vi "HW_Gantner_Search Devices in System.vi"(8 "error in":errorcluster caption="错误输入") -> (0 "error out":errorcluster caption="错误输出", 1 "Modu[] info":T7[](array[typedef]), 3 "Configuration out":T1 {"StartTime" format="%#.10f"; "dActTimeToSecondFactor" format="%#.10f"; "StartTimeToDayFactor" format="%#_10f"})   [LabVIEW 2016]
doc: "检测系统中的NI设备：\n包括机箱信息、模块信息、通道基本信息等。\n\n两种方式：\n1、配置文件中读取\n2、自动检测\n具体实现方式在配置文件中配置。"
uses:
  Gantner Device Info.ctl
  GantnerDriver/Gantner-Instruments HighSpeedPort/e.gate Configuration.ctl
  GantnerDriver/Gantner-Instruments HighSpeedPort/e.gate Channel Data.ctl
  GantnerDriver/Gantner-Instruments HighSpeedPort/e.gate Data Type.ctl
  GantnerDriver/Gantner-Instruments HighSpeedPort/e.gate Protocol Type.ctl
  GantnerDriver/Gantner-Instruments HighSpeedPort/e.gate Module  Data.ctl
  GantnerDriver/Gantner-Instruments HighSpeedPort/e.gateHSP_DLLhandle.ctl
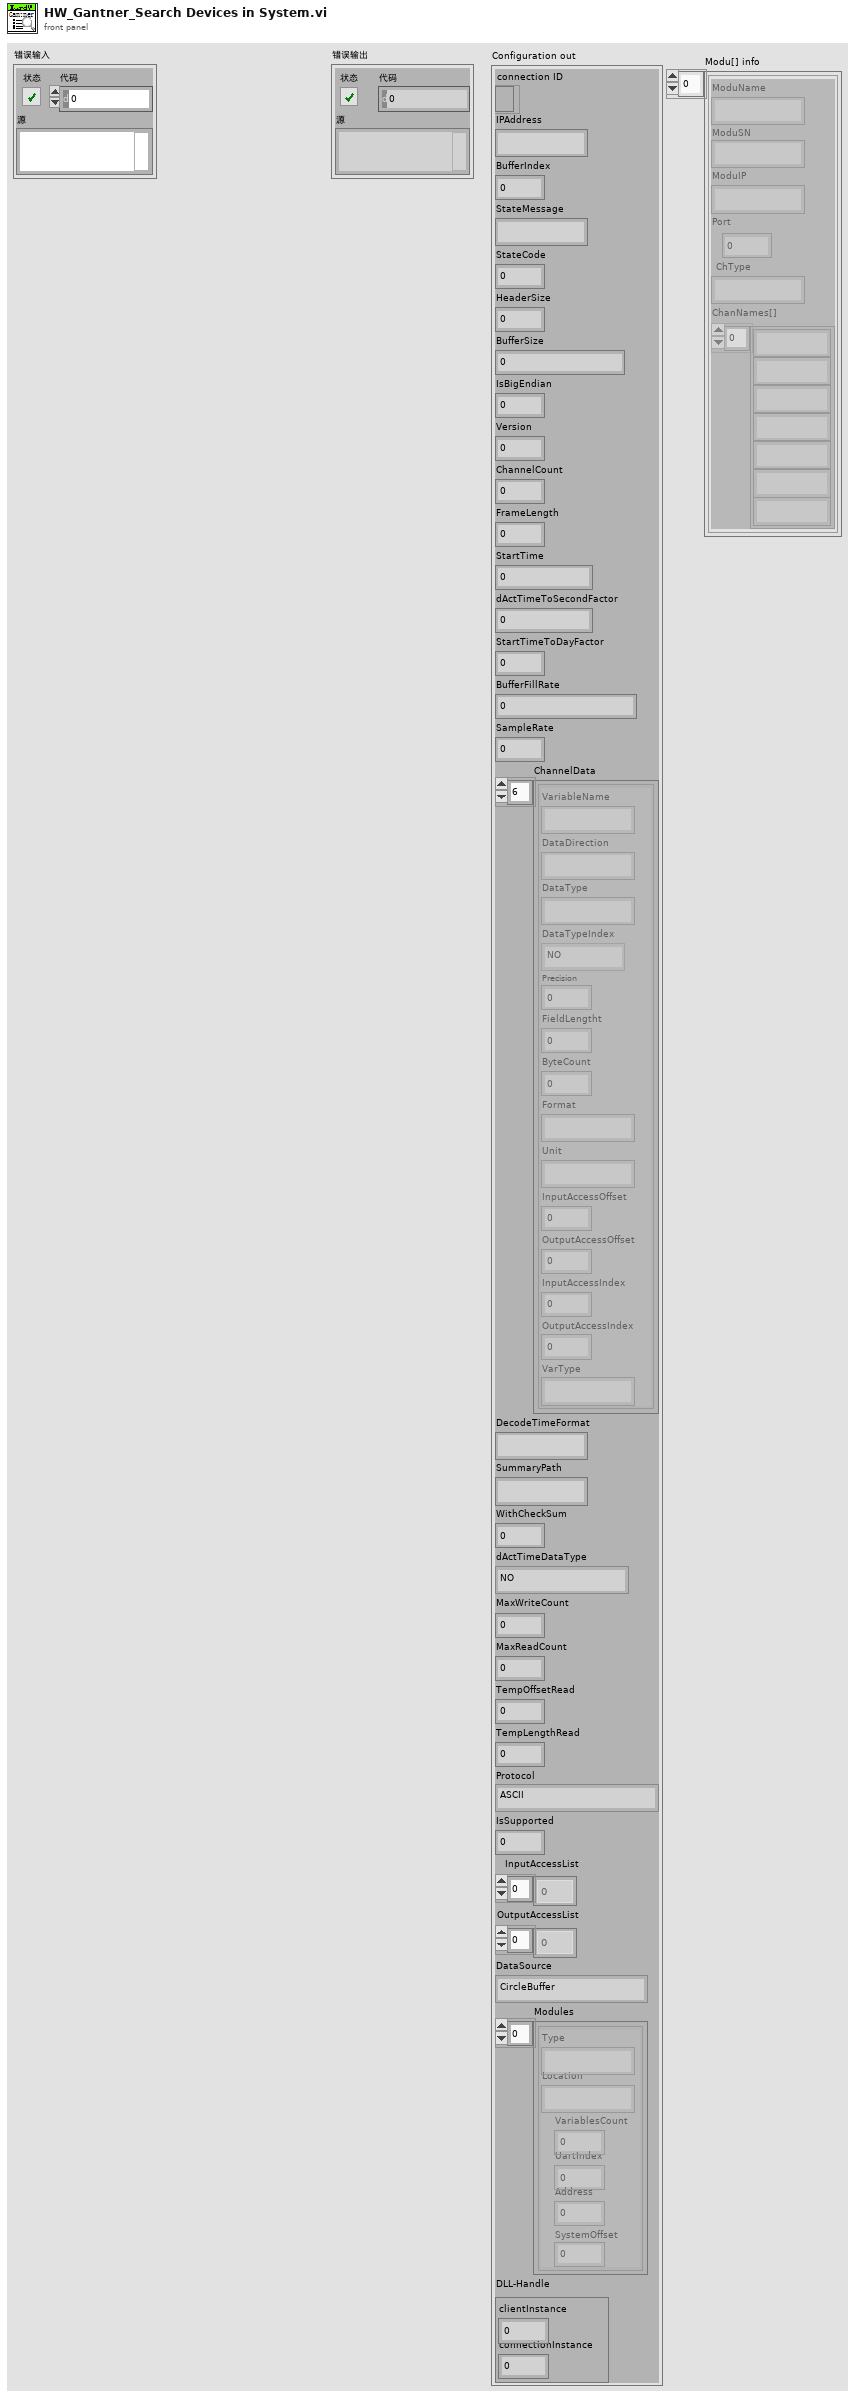
[diagram p1: front panel]
types:
  T1 = typedef "e.gate Configuration.ctl" = cluster{"connection ID":refnum<k5>, "IPAddress":string, "BufferIndex":i32, "StateMessage":string, "StateCode":i8, "HeaderSize":i32, "BufferSize":i32, "IsBigEndian":i32, "Version":i32, "ChannelCount":i32, "FrameLength":i32, "StartTime":dbl, "dActTimeToSecondFactor":dbl, "StartTimeToDayFactor":dbl, "BufferFillRate":dbl, "SampleRate":dbl, "ChannelData":T2[], "DecodeTimeFormat":string, "SummaryPath":string, "WithCheckSum":i32, "dActTimeDataType":T3, "MaxWriteCount":i32, "MaxReadCount":i32, "TempOffsetRead":i32, "TempLengthRead":i32, "Protocol":T4, "IsSupported":i32, "InputAccessList":i32[], "OutputAccessList":i32[], "DataSource":enum16{"CircleBuffer", "test.con Logger", "test.con Archive"}, "Modules":T5[], "DLL-Handle":T6}
  T2 = typedef "e.gate Channel Data.ctl" = cluster{"VariableName":string, "DataDirection":string, "DataType":string, "DataTypeIndex":T3, "Precision":i16, "FieldLengtht":i16, "ByteCount":i32, "Format":string, "Unit":string, "InputAccessOffset":i32, "OutputAccessOffset":i16, "InputAccessIndex":i16, "OutputAccessIndex":i16, "VarType":string}
  T3 = typedef "e.gate Data Type.ctl" = enum16{"NO", "BOOL", "SINT8", "USINT8", "SINT16", "USINT16", "SINT32", "USINT32", "FLOAT", "SET8", "SET16", "SET32", "DOUBLE", "SINT64", "USINT64", "SET64"}
  T4 = typedef "e.gate Protocol Type.ctl" = enum16{"ASCII", "HighspeedPort Online", "HighspeedPort Buffer", "eGateHighspeedPortDLL "}
  T5 = typedef "e.gate Module  Data.ctl" = cluster{"Type":string, "Location":string, "VariablesCount":i16, "UartIndex":i16, "Address":i16, "SystemOffset":i16}
  T6 = typedef "e.gateHSP_DLLhandle.ctl" = cluster{"clientInstance":i32, "connectionInstance":i32}
  T7 = typedef "Gantner Device Info.ctl" = cluster{"ModuName":string, "ModuSN":string, "ModuIP":string, "Port":i32, "ChType":string, "ChanNames[]":string[]}
  T8 = enum16{"CircleBuffer", "test.con Logger", "test.con Archive"}
  T9 = cluster{"Type":string, "Location":string, "Vendor":string, "MKCode":string, "DHCPMode":string, "IPAddress":string, "SubnetMask":string, "GatewayAddress":string, "MACAddress":string, "SerialNumber":string}[]
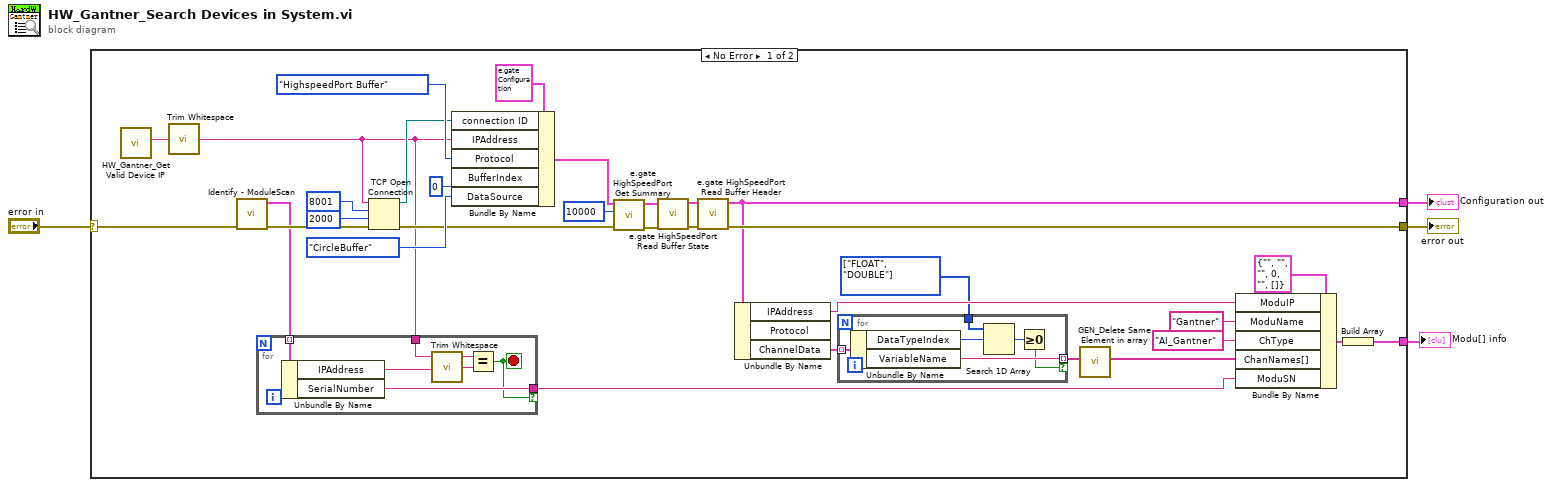
[diagram p0: block diagram]
diagram:
  n1 = case shown="No Error" "error in" {
    selector: "error in" -> [w14 w49]
    tunnel: [w10 w49] -> w3
    tunnel: [w17 _] -> w2
    tunnel: [w8 _] -> w1
    frame No Error {
      w5 = T3[] [enum."FLOAT", enum."DOUBLE"] items=["NO", "BOOL", "SINT8", "USINT8", "SINT16", "USINT16", "SINT32", "USINT32", "FLOAT", "SET8", "SET16", "SET32", "DOUBLE", "SINT64", "USINT64", "SET64"]
      n2 = call "HW_Gantner_Get Valid Device IP.vi"() -> ("ip out"=w22:string)  [unwired: 11 in]
      n3 = call <vilib>:"Trim Whitespace.vi"("string"=w22) -> ("trimmed string"=w9:string)  [unwired: 1 in]
      n4 = call "Identify - ModuleScan.vi"("Fehler (Eingang, kein Fehler)"=w14) -> ("Fehler (Ausgang)"=w13:errorcluster, "LifeList"=w12:T9)  [unwired: 9 in]
      n5 = for {
        tunnel: w12 -> [w42] mode=indexing
        tunnel: w9 -> [w41]
        tunnel: [w40] -> w11 if=w39
        stop <- w39 stop-if-true
        n6 = Unbundle By Name(w42) -> ("IPAddress"=w38:string, "SerialNumber"=w40:string)
        n7 = call <vilib>:"Trim Whitespace.vi"("string"=w38) -> ("trimmed string"=w37:string)  [unwired: 1 in]
        n8 = Equal?(x=w41, y=w37) -> (x = y?=w39:bool)
      }
      n9 = TCP Open Connection(address=w9, remote port or service name=u16 8001, timeout ms (60000)=2000 ("Timeout in ms (60000)"), error in (no error)=w13) -> (connection ID=w23:refnum<k5>, error out=w26:errorcluster)  [unwired: 1 out]
      n10 = Bundle By Name(cluster=T1 {"connection ID"=refnum, "IPAddress"="", "BufferIndex"=0, "StateMessage"="", "StateCode"=0, "HeaderSize"=0, "BufferSize"=0, "IsBigEndian"=0, "Version"=0, "ChannelCount"=0, "FrameLength"=0, "StartTime"=0.0, "dActTimeToSecondFactor"=0.0, "StartTimeToDayFactor"=0.0, "BufferFillRate"=0.0, "SampleRate"=0.0, "ChannelData"=[], "DecodeTimeFormat"="", "SummaryPath"="", "WithCheckSum"=0, "dActTimeDataType"=enum."NO", "MaxWriteCount"=0, "MaxReadCount"=0, "TempOffsetRead"=0, "TempLengthRead"=0, "Protocol"=enum."ASCII", "IsSupported"=0, "InputAccessList"=[], "OutputAccessList"=[], "DataSource"=enum."CircleBuffer", "Modules"=[], "DLL-Handle"={"clientInstance"=0, "connectionInstance"=0}} ("e.gate Configuration"), "connection ID"=w23, "IPAddress"=w9, "Protocol"=e.gate_Protocol_Type."HighspeedPort Buffer", "BufferIndex"=0, "DataSource"=T8."CircleBuffer") -> (w24:T1)
      n11 = call "e.gate HighSpeedPort Get Summary.vi"("error in (no error)"=w26, "Timeout (ms) [1000]"=10000, "Configuration in"=w24) -> ("error out"=w34:errorcluster, "Configuration out"=w35:T1)  [unwired: 7 out]
      n12 = call "e.gate HighSpeedPort Read Buffer State.vi"("error in (no error)"=w34, "Configuration in"=w35) -> ("Error out"=w32:errorcluster, "Configuration out"=w33:T1)  [unwired: 8 out]
      n13 = call "e.gate HighSpeedPort Read Buffer Header.vi"("error in (no error)"=w32, "Configuration in"=w33) -> ("error out"=w10:errorcluster, "Configuration out"=w8:T1)  [unwired: 8 out]
      n14 = Unbundle By Name(w8) -> ("IPAddress"=w16:string, "ChannelData"=w21:T2[])  [unwired: 1 out]
      n15 = for {
        tunnel: w21 -> [w48] mode=indexing
        tunnel: [w47] -> w7 mode=indexing if=w43
        tunnel: w5 -> [w46]
        n16 = Unbundle By Name(w48) -> ("DataTypeIndex"=w45:T3, "VariableName"=w47:string)
        n17 = Search 1D Array(1D array=w46, element=w45) -> (index of element=w44:i32)  [unwired: 1 in]
        n18 = Greater Or Equal To 0?(x=w44) -> (x >= 0?=w43:bool)
      }
      n19 = call "GEN_Delete Same Element in array.vi"("data in"=w7) -> ("data out"=w6:string[])  [unwired: 10 in]
      n20 = Bundle By Name(cluster=T7 {"ModuName"="", "ModuSN"="", "ModuIP"="", "Port"=0, "ChType"="", "ChanNames[]"=[]} ("DevInfo"), "ModuIP"=w16, "ModuName"="Gantner" ("ModName"), "ChType"="AI_Gantner" ("ChanInfo.ChanType"), "ChanNames[]"=w6, "ModuSN"=w11) -> (w18:T7)
      n21 = Build Array(w18) -> (w17:T7[])
    }
    frame Error {
    }
  }
  "error out" <- w3
  "Modu[] info" <- w2
  "Configuration out" <- w1
